vi "VisualizeModulePositioning_standalone.vi"() -> ()   [LabVIEW 2016]
uses:
  2_ModulePositioning/SingleModuleProgressReport.ctl
  <vilib>/vision/driver/NI_Vision_Acquisition_Software.lvlib
  <vilib>/vision/NI_Vision_Development_Module.lvlib
panel:
  in  "Placement tolerance [um]":dbl=10.0
  in  "Calibration [um/pix]":dbl=0.25
  out "delta Y":sgl
  out "delta X":sgl
  out "Current Position":T1
  in  "Axis Speeds":T2={"X [mm/s]"=25.0, "Y [mm/s]"=12.5, "Z [mm/s]"=5.0}
  in  "stop":bool
  out "Placement Monitor":T3(plugin-control)
  out "Fiducial Template":T3(plugin-control)
  in  "Templates path":path=path "C:/Users/Aerotech/Documents/BNL_ThermomechanicalStave"
  in  "Module fiducial marker":T4(ring)=enum."[None]"
  out "Module Progress Report":T5(array[cluster])
  in  "Camera Name":refnum<k21>="cam0" caption="IMAQdx Session"
  in  "N modules":i32
  in  "Calibrated positions of fiducials [mm]":dbl[][](array[numeric])=[[-675.4228165149058, -196.82430550413875, -11.55], [-579.8428201474238, -196.8506568257386, -11.55], [-579.816468825824, -101.27066045825673, -11.55], [-675.3964651933059, -101.24430913665685, -11.55], [-577.422820239396, -196.8513240176017, -11.55], [-481.84282387191405, -196.87767533920157, -11.55], [-481.8164725503142, -101.29767897171968, -11.55], [-577.396468917796, -101.2713276501198, -11.55], [-479.42282396388623, -196.87834253106465, -11.55], [-383.8428275964043, -196.90469385266454, -11.55], [-383.81647627480436, -101.32469748518264, -11.55], [-479.3964726422863, -101.29834616358275, -11.55], [-381.42282768837646, -196.90536104452758, -11.55], [-285.8428313208945, -196.93171236612747, -11.55], [-285.8164799992946, -101.35171599864559, -11.55], [-381.39647636677654, -101.3253646770457, -11.55], [-283.4228314128667, -196.93237955799054, -11.55], [-187.84283504538473, -196.95873087959043, -11.55], [-187.8164837237848, -101.37873451210854, -11.55], [-283.39648009126677, -101.35238319050865, -11.55], [-185.42283513735697, -196.9593980714535, -11.55], [-89.84283876987502, -196.98574939305337, -11.55], [-89.81648744827521, -101.40575302557149, -11.55], [-185.39648381575705, -101.3794017039716, -11.55], [-87.42283886184703, -196.98641658491644, -11.55], [8.157157505634814, -197.01276790651633, -11.55], [8.183508827234618, -101.43277153903443, -11.55], [-87.39648754024722, -101.40642021743454, -11.55], [10.57715741366269, -197.01343509837938, -11.55], [106.15715378114453, -197.0397864199793, -11.55], [106.18350510274433, -101.45979005249738, -11.55], [10.603508735262494, -101.4334387308975, -11.55], [108.57715368917252, -197.04045361184234, -11.55], [204.15715005665436, -197.06680493344223, -11.55], [204.18350137825416, -101.48680856596033, -11.55], [108.60350501077232, -101.46045724436046, -11.55], [206.57714996468223, -197.0674721253053, -11.55], [302.1571463321641, -197.09382344690516, -11.55], [302.1834976537639, -101.5138270794233, -11.55], [206.60350128628204, -101.4874757578234, -11.55], [304.57714624019206, -197.09449063876826, -11.55], [400.1571426076739, -197.12084196036813, -11.55], [400.1834939292737, -101.54084559288623, -11.55], [304.60349756179187, -101.51449427128635, -11.55], [402.5771425157018, -197.1215091522312, -11.55], [498.15713888318373, -197.1478604738311, -11.55], [498.18349020478354, -101.56786410634919, -11.55], [402.6034938373016, -101.5415127847493, -11.55], [500.5771387912116, -197.14852766569413, -11.55], [596.1571351586933, -197.17487898729405, -11.55], [596.1834864802931, -101.59488261981214, -11.55], [500.6034901128114, -101.56853129821225, -11.55]]
  # "-101.244"
  # "-196.851"
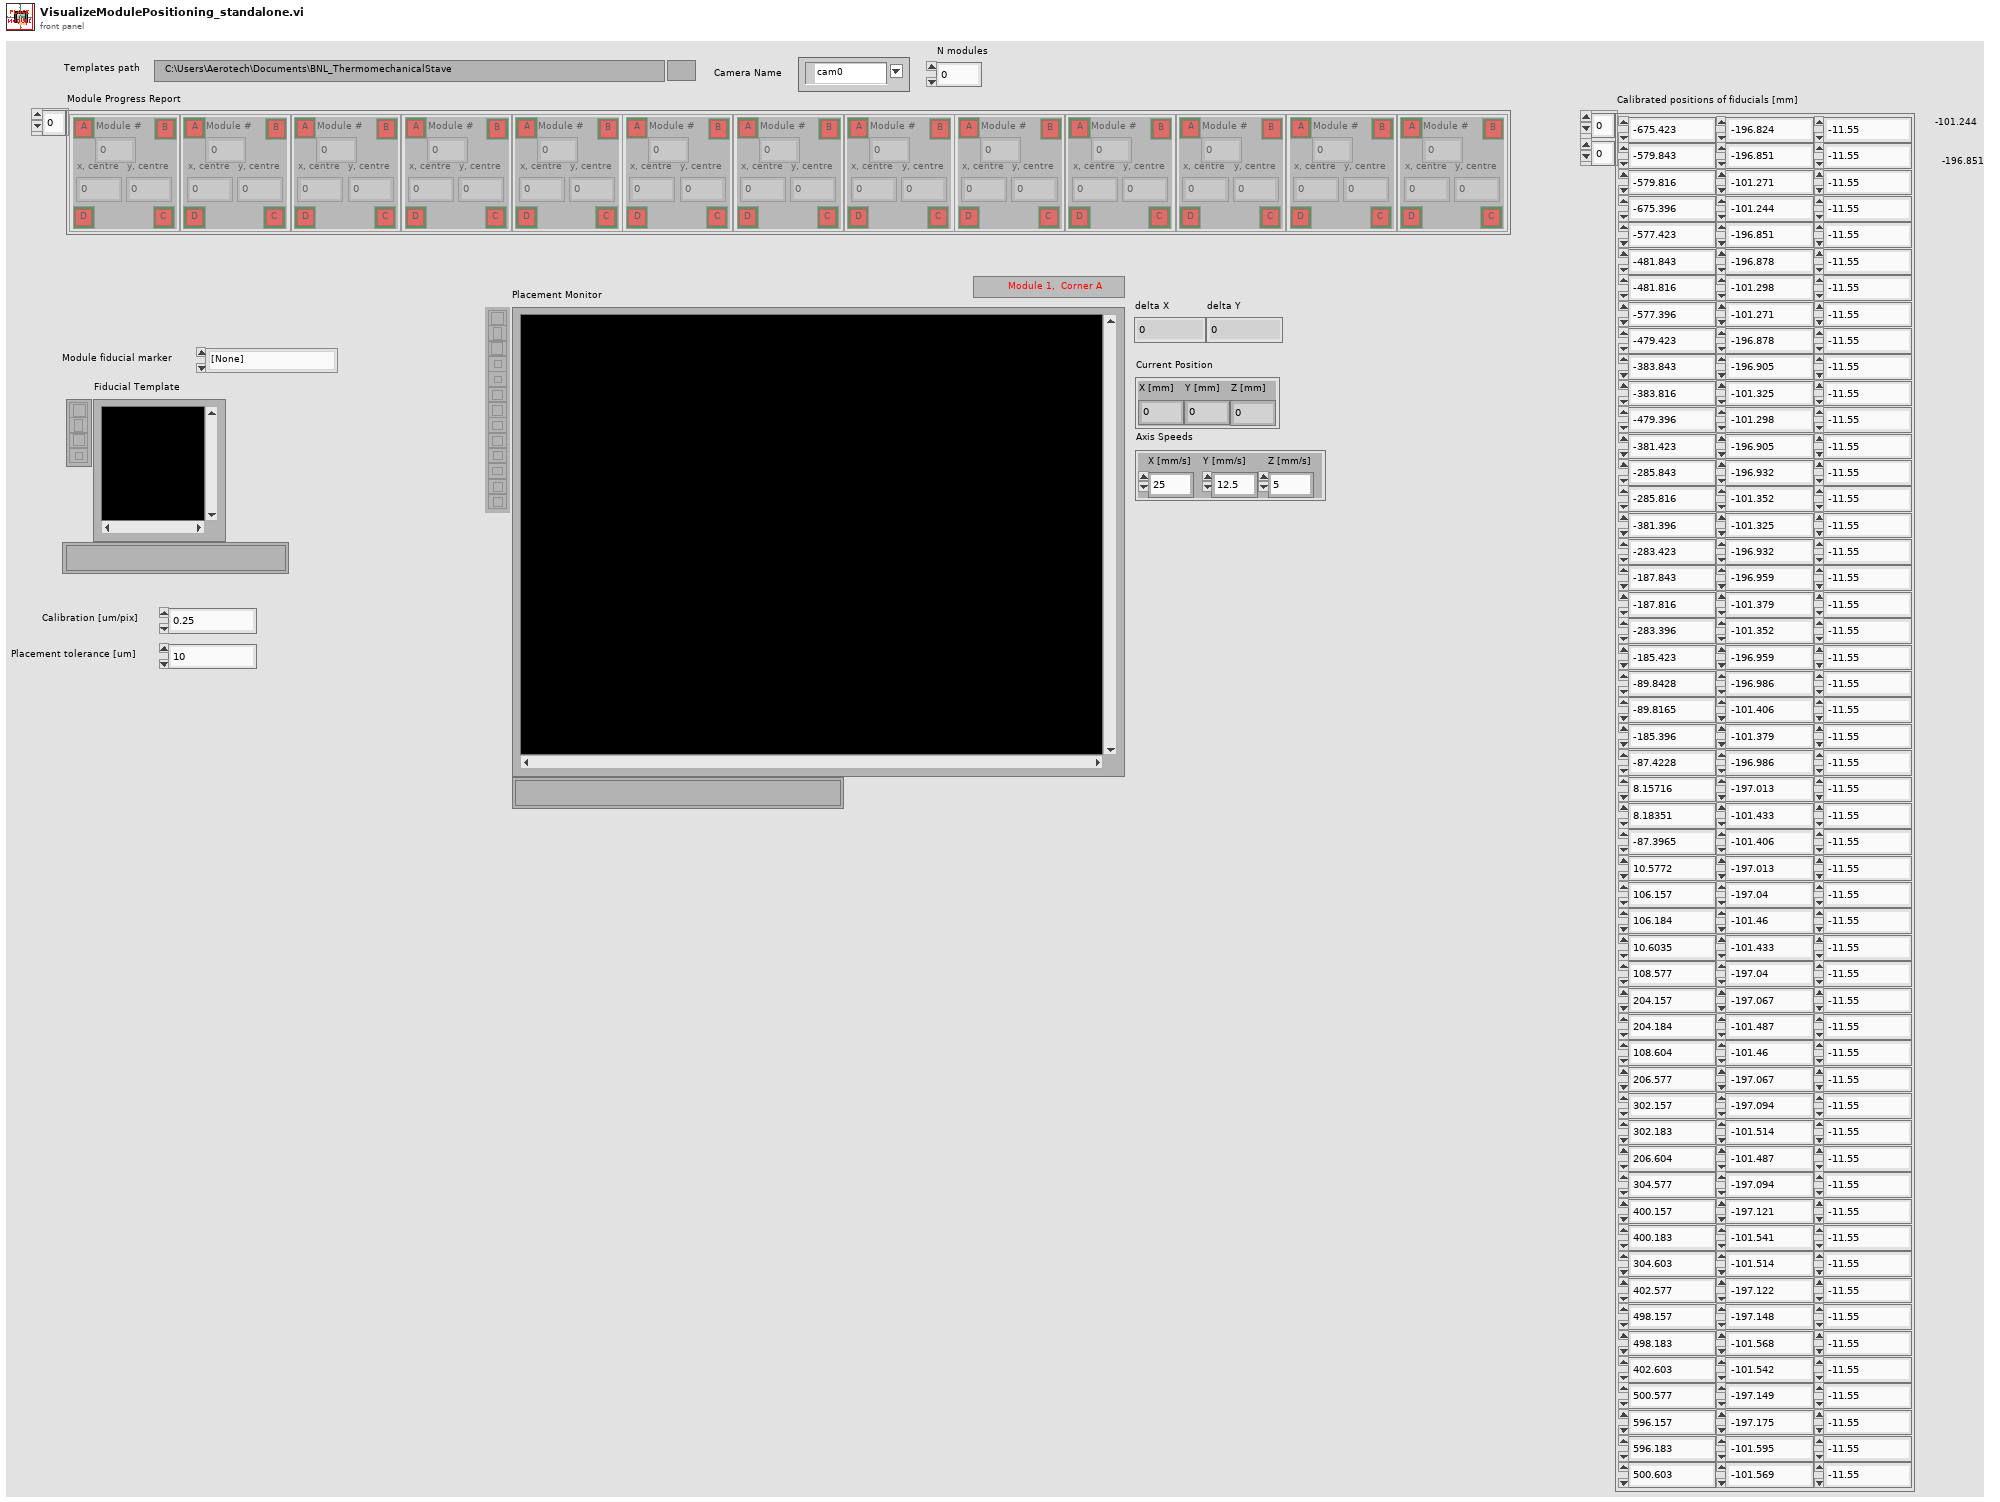
[diagram p1: front panel]
types:
  T1 = cluster{"X [mm]":dbl, "Y [mm]":dbl, "Z [mm]":dbl}
  T2 = cluster{"X [mm/s]":dbl, "Y [mm/s]":dbl, "Z [mm/s]":dbl}
  T3 = typedef "IMAQ Image.ctl" = refnum<image>
  T4 = enum16{"Mark C", "Mark B", "Strip Corner", "[None]"}
  T5 = cluster{"A":bool, "x, centre":dbl, "y, centre":dbl, "Module #":i32, "B":bool, "D":bool, "C":bool}[]
  T6 = typedef "SingleModuleProgressReport.ctl" = cluster{"A":bool, "x, centre":dbl, "y, centre":dbl, "Module #":i32, "B":bool, "D":bool, "C":bool}
  T7 = cluster{"Algorithm":i32, "Number of Matches Requested":i32, "Minimum Match Score":sgl, "SubPixel Accuracy":bool, "Rotation Angle Ranges":cluster{"Start":sgl, "End":sgl}[], "Show Search Area":bool, "Show Result":bool}
  T8 = typedef "IMAQdx.ctl" = refnum<k21>
  T9 = cluster{"Final X":dbl, "Final Y":dbl, "Final Z":dbl}
  T10 = cluster{"Position":cluster{"x":sgl, "y":sgl}, "Angle":sgl, "Scale":sgl, "Score":sgl, "Bounding Box":cluster{"x":sgl, "y":sgl}[]}[]
  T11 = cluster{"Position":cluster{"x":sgl, "y":sgl}, "Angle":sgl, "Scale":sgl, "Score":sgl, "Bounding Box":cluster{"x":sgl, "y":sgl}[]}
  T12 = cluster{"A":bool, "x, centre":dbl, "y, centre":dbl, "Module #":i32, "B":bool, "D":bool, "C":bool}
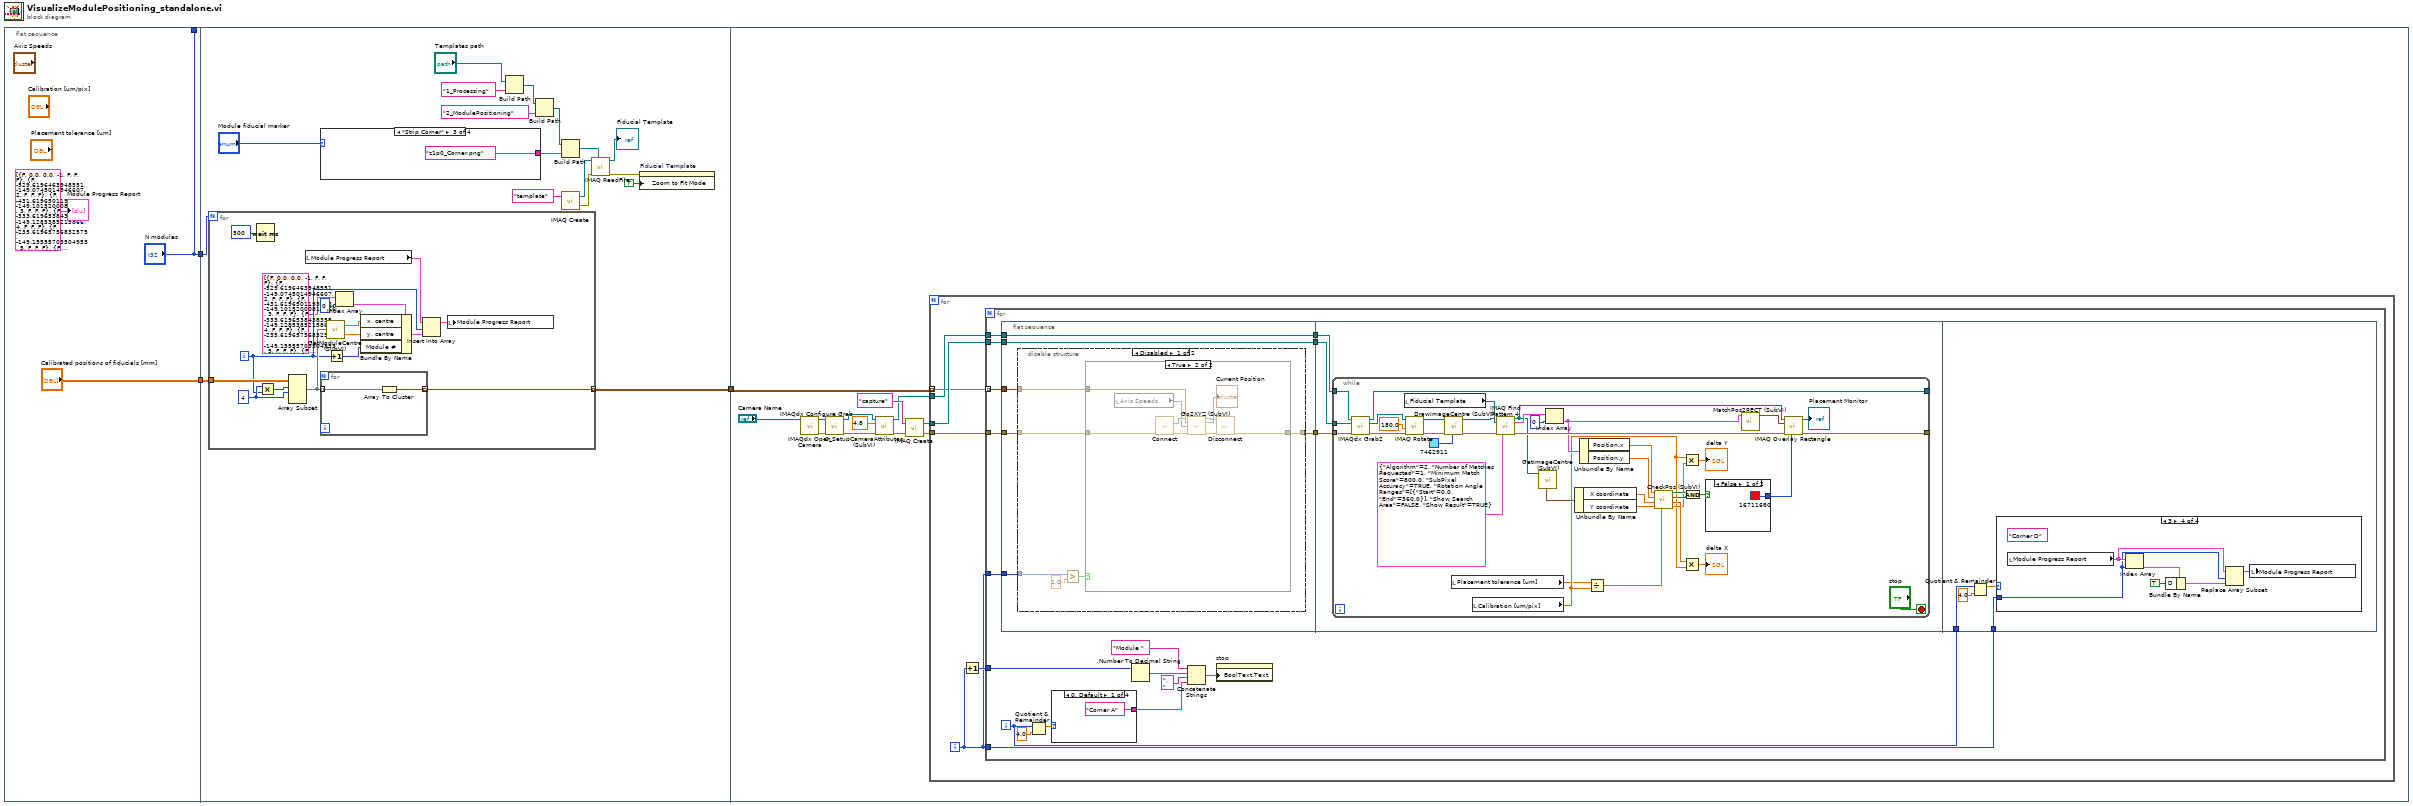
[diagram p0: block diagram]
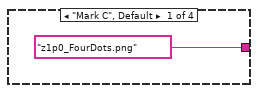
[diagram p2: hidden frame]
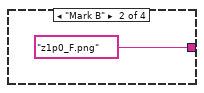
[diagram p3: hidden frame]
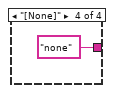
[diagram p4: hidden frame]
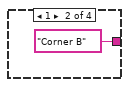
[diagram p5: hidden frame]
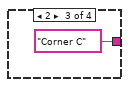
[diagram p6: hidden frame]
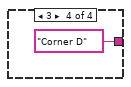
[diagram p7: hidden frame]
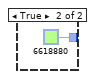
[diagram p10: hidden frame]
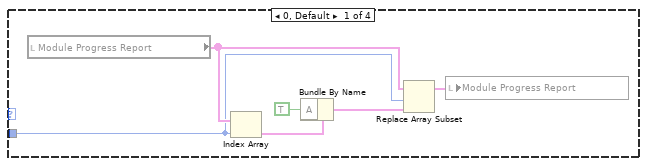
[diagram p11: hidden frame]
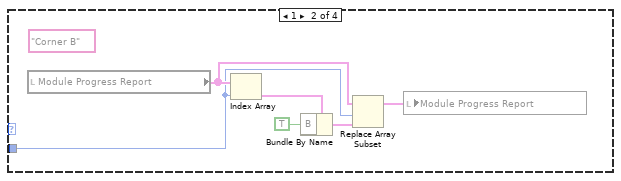
[diagram p12: hidden frame]
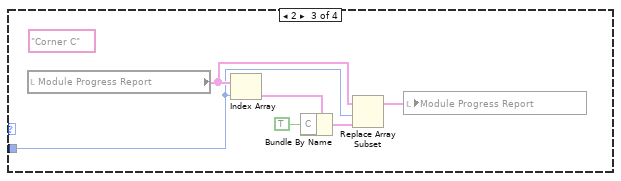
[diagram p13: hidden frame]
diagram:
  n1 = flat-sequence {
    tunnel: ["N modules"] -> _
    tunnel: ["N modules"] -> w2
    tunnel: ["Calibrated positions of fiducials [mm]"] -> w1
    tunnel: [w21] -> w3
    tunnel: w2 -> [w23]
    tunnel: w1 -> [w22]
    tunnel: w3 -> [w46]
    frame #0 {
      "Module Progress Report" <- T6[] [{"A"=FALSE, "x, centre"=0.0, "y, centre"=0.0, "Module #"=-1, "B"=FALSE, "D"=FALSE, "C"=FALSE}, {"A"=FALSE, "x, centre"=-529.6196463948551, "y, centre"=-149.0745014946607, "Module #"=2, "B"=FALSE, "D"=FALSE, "C"=FALSE}, {"A"=FALSE, "x, centre"=-431.6196501193453, "y, centre"=-149.10152000812366, "Module #"=3, "B"=FALSE, "D"=FALSE, "C"=FALSE}, {"A"=FALSE, "x, centre"=-333.6196538438355, "y, centre"=-149.1285385215866, "Module #"=4, "B"=FALSE, "D"=FALSE, "C"=FALSE}, {"A"=FALSE, "x, centre"=-235.61965756832575, "y, centre"=-149.15555703504953, "Module #"=5, "B"=FALSE, "D"=FALSE, "C"=FALSE}, {"A"=FALSE, "x, centre"=-137.6196612928161, "y, centre"=-149.1825755485125, "Module #"=6, "B"=FALSE, "D"=FALSE, "C"=FALSE}, {"A"=FALSE, "x, centre"=-627.6196426703649, "y, centre"=-149.04748298119773, "Module #"=1, "B"=FALSE, "D"=FALSE, "C"=FALSE}, {"A"=FALSE, "x, centre"=-529.6196463948551, "y, centre"=-149.0745014946607, "Module #"=2, "B"=FALSE, "D"=FALSE, "C"=FALSE}, {"A"=FALSE, "x, centre"=-431.6196501193453, "y, centre"=-149.10152000812366, "Module #"=3, "B"=FALSE, "D"=FALSE, "C"=FALSE}, {"A"=FALSE, "x, centre"=-333.6196538438355, "y, centre"=-149.1285385215866, "Module #"=4, "B"=FALSE, "D"=FALSE, "C"=FALSE}, {"A"=FALSE, "x, centre"=-235.61965756832575, "y, centre"=-149.15555703504953, "Module #"=5, "B"=FALSE, "D"=FALSE, "C"=FALSE}, {"A"=FALSE, "x, centre"=-137.6196612928161, "y, centre"=-149.1825755485125, "Module #"=6, "B"=FALSE, "D"=FALSE, "C"=FALSE}, {"A"=FALSE, "x, centre"=-39.619665017306204, "y, centre"=-149.20959406197545, "Module #"=7, "B"=FALSE, "D"=FALSE, "C"=FALSE}, {"A"=FALSE, "x, centre"=58.38033125820351, "y, centre"=-149.2366125754384, "Module #"=8, "B"=FALSE, "D"=FALSE, "C"=FALSE}, {"A"=FALSE, "x, centre"=156.38032753371334, "y, centre"=-149.26363108890132, "Module #"=9, "B"=FALSE, "D"=FALSE, "C"=FALSE}, {"A"=FALSE, "x, centre"=254.38032380922306, "y, centre"=-149.29064960236428, "Module #"=10, "B"=FALSE, "D"=FALSE, "C"=FALSE}, {"A"=FALSE, "x, centre"=352.3803200847329, "y, centre"=-149.31766811582725, "Module #"=11, "B"=FALSE, "D"=FALSE, "C"=FALSE}, {"A"=FALSE, "x, centre"=450.38031636024266, "y, centre"=-149.3446866292902, "Module #"=12, "B"=FALSE, "D"=FALSE, "C"=FALSE}, {"A"=FALSE, "x, centre"=548.3803126357524, "y, centre"=-149.37170514275314, "Module #"=13, "B"=FALSE, "D"=FALSE, "C"=FALSE}] ("Module Progress Report")
    }
    frame #1 {
      n2 = for {
        N: w23 -> [_]
        tunnel: w22 -> [w43]
        tunnel: [w40] -> w21 mode=indexing
        i -> [w31]
        w41 = 4 ("x")
        n3 = Wait (ms)(milliseconds to wait=u32 500) -> ()  [unwired: 1 out]
        n4 = Multiply(x=w41, y=w31) -> (x*y=w42:i32)
        n5 = Array Subset(array=w43, index (row)=w42, length (row)=w41) -> (w39:dbl[][])  [unwired: 2 in]
        n6 = local read "Module Progress Report"() -> (w32:T5)
        n7 = for {
          tunnel: w39 -> [w44] mode=indexing
          tunnel: [w45] -> w40 mode=indexing
          n8 = Array To Cluster(array=w44) -> (cluster=w45:cluster{"[0]":dbl, "[1]":dbl, "[2]":dbl})
        }
        n9 = call "GetModuleCentre (SubVI).vi"("4x3 Array of Fiducial Coordinates"=w39) -> ("x, centre"=w38:dbl, "y, centre"=w37:dbl)
        n10 = Increment(x=w31) -> (x+1=w36:i32)
        n11 = Index Array(array=T6[] [{"A"=FALSE, "x, centre"=0.0, "y, centre"=0.0, "Module #"=-1, "B"=FALSE, "D"=FALSE, "C"=FALSE}, {"A"=FALSE, "x, centre"=-529.6196463948551, "y, centre"=-149.0745014946607, "Module #"=2, "B"=FALSE, "D"=FALSE, "C"=FALSE}, {"A"=FALSE, "x, centre"=-431.6196501193453, "y, centre"=-149.10152000812366, "Module #"=3, "B"=FALSE, "D"=FALSE, "C"=FALSE}, {"A"=FALSE, "x, centre"=-333.6196538438355, "y, centre"=-149.1285385215866, "Module #"=4, "B"=FALSE, "D"=FALSE, "C"=FALSE}, {"A"=FALSE, "x, centre"=-235.61965756832575, "y, centre"=-149.15555703504953, "Module #"=5, "B"=FALSE, "D"=FALSE, "C"=FALSE}, {"A"=FALSE, "x, centre"=-137.6196612928161, "y, centre"=-149.1825755485125, "Module #"=6, "B"=FALSE, "D"=FALSE, "C"=FALSE}, {"A"=FALSE, "x, centre"=-627.6196426703649, "y, centre"=-149.04748298119773, "Module #"=1, "B"=FALSE, "D"=FALSE, "C"=FALSE}, {"A"=FALSE, "x, centre"=-529.6196463948551, "y, centre"=-149.0745014946607, "Module #"=2, "B"=FALSE, "D"=FALSE, "C"=FALSE}, {"A"=FALSE, "x, centre"=-431.6196501193453, "y, centre"=-149.10152000812366, "Module #"=3, "B"=FALSE, "D"=FALSE, "C"=FALSE}, {"A"=FALSE, "x, centre"=-333.6196538438355, "y, centre"=-149.1285385215866, "Module #"=4, "B"=FALSE, "D"=FALSE, "C"=FALSE}, {"A"=FALSE, "x, centre"=-235.61965756832575, "y, centre"=-149.15555703504953, "Module #"=5, "B"=FALSE, "D"=FALSE, "C"=FALSE}, {"A"=FALSE, "x, centre"=-137.6196612928161, "y, centre"=-149.1825755485125, "Module #"=6, "B"=FALSE, "D"=FALSE, "C"=FALSE}, {"A"=FALSE, "x, centre"=-39.619665017306204, "y, centre"=-149.20959406197545, "Module #"=7, "B"=FALSE, "D"=FALSE, "C"=FALSE}, {"A"=FALSE, "x, centre"=58.38033125820351, "y, centre"=-149.2366125754384, "Module #"=8, "B"=FALSE, "D"=FALSE, "C"=FALSE}, {"A"=FALSE, "x, centre"=156.38032753371334, "y, centre"=-149.26363108890132, "Module #"=9, "B"=FALSE, "D"=FALSE, "C"=FALSE}, {"A"=FALSE, "x, centre"=254.38032380922306, "y, centre"=-149.29064960236428, "Module #"=10, "B"=FALSE, "D"=FALSE, "C"=FALSE}, {"A"=FALSE, "x, centre"=352.3803200847329, "y, centre"=-149.31766811582725, "Module #"=11, "B"=FALSE, "D"=FALSE, "C"=FALSE}, {"A"=FALSE, "x, centre"=450.38031636024266, "y, centre"=-149.3446866292902, "Module #"=12, "B"=FALSE, "D"=FALSE, "C"=FALSE}, {"A"=FALSE, "x, centre"=548.3803126357524, "y, centre"=-149.37170514275314, "Module #"=13, "B"=FALSE, "D"=FALSE, "C"=FALSE}] ("Module Progress Report"), index=0) -> (element=w33:T6)
        n12 = Bundle By Name(cluster=w33, "x, centre"=w38, "y, centre"=w37, "Module #"=w36) -> (w28:T6)
        n13 = Insert Into Array(array=w32, index=w31, new element=w28) -> (w30:T5)
        n14 = local write "Module Progress Report"(w30) -> ()
      }
      n15 = case shown="\"Strip Corner\"" "Module fiducial marker" {
        tunnel: ["z1p0_FourDots.png" ("name or relative path") "z1p0_F.png" ("name or relative path") "z1p0_Corner.png" ("name or relative path") "none" ("name or relative path")] -> w20
        frame "Mark C", Default {
        }
        frame "Mark B" {
        }
        frame "Strip Corner" {
        }
        frame "[None]" {
        }
      }
      n16 = Build Path(base path="Templates path", name or relative path="1_Processing") -> (appended path=w7:path)
      n17 = Build Path(base path=w7, name or relative path="2_ModulePositioning") -> (appended path=w18:path)
      n18 = Build Path(base path=w18, name or relative path=w20) -> (appended path=w17:path)
      n19 = call "IMAQ Create"("Image Name"="template") -> ("New Image"=w16:T3, "error out"=w15:errorcluster)  [unwired: 4 in]
      n20 = call "IMAQ ReadFile"("File Path"=w17, "error in (no error)"=w15, "Image"=w16) -> ("error out"=w11:errorcluster, "Image Out"=→"Fiducial Template":T3)  [unwired: 4 in, 3 out]
      n21 = property on="Fiducial Template" class="ImageControl"(error in=w11, "Zoom to Fit Mode"=TRUE) -> ()  [unwired: 1 in, 2 out]
    }
    frame #2 {
      n22 = call <vilib>:"IMAQdx Open Camera.vi"("Session In"="Camera Name") -> ("error out"=w55:errorcluster, "Session Out"=w56:T8)  [unwired: 2 in, 7 out]
      n23 = call <vilib>:"IMAQdx Configure Grab.vi"("error in"=w55, "Session In"=w56) -> ("error out"=w53:errorcluster, "Session Out"=w54:T8)  [unwired: 8 out]
      n24 = call "0_SetupCameraAttributes (SubVI).vi"("error in (no error)"=w53, "Gain"=4.8, "Camera session in"=w54) -> ("error out"=w51:errorcluster, "Camera session out"=w48:T8)  [unwired: 7 in]
      n25 = call "IMAQ Create"("Image Name"="capture", "error in (no error)"=w51) -> ("New Image"=w49:T3, "error out"=w47:errorcluster)  [unwired: 3 in]
      n26 = for {
        tunnel: w48 -> [w63]
        tunnel: w49 -> [w62]
        tunnel: w47 -> [w61]
        tunnel: w46 -> [w59] mode=indexing
        i -> [w58]
        n27 = Increment(x=w58) -> (x+1=w60:i32)
        n28 = for {
          tunnel: w63 -> [w78]
          tunnel: w62 -> [w77]
          tunnel: w61 -> [w76]
          tunnel: w60 -> [w71]
          tunnel: w59 -> [w67] mode=indexing
          tunnel: w58 -> [w66]
          tunnel: w58 -> [w64]
          i -> [w65]
          n29 = flat-sequence {
            tunnel: w78 -> [w90]
            tunnel: w76 -> [w89]
            tunnel: w77 -> [w91]
            tunnel: [w91] -> w81
            tunnel: [w88] -> w80
            tunnel: [w90] -> w79
            tunnel: w67 -> [w87]
            tunnel: w64 -> [w86]
            tunnel: w81 -> [w110]
            tunnel: w80 -> [w109]
            tunnel: w79 -> [w108]
            tunnel: w66 -> [w153]
            tunnel: w65 -> [w152]
            frame #0 {
              n30 = disable-structure shown="Disabled" {
                disable-tunnel: w89 -> [w97 _]
                disable-tunnel: [w96 _] -> w88
                disable-tunnel: w87 -> [w95 _]
                disable-tunnel: w86 -> [w92 _]
                frame Disabled {
                  n31 = Greater?(x=w92, y=1.0) -> (0:w94:bool)
                  n32 = case shown="True" w94 {
                    tunnel: w97 -> [w98 w107]
                    tunnel: [w98 w106] -> w96
                    tunnel: w95 -> [_ w105]
                    frame False {
                      # "Temporarily skip corners C and D"
                    }
                    frame True {
                      n33 = local read "Axis Speeds"() -> (w99:T2)
                      n34 = call "Connect.vi"("error in (no error)"=w107) -> ("error out"=w103:errorcluster, "controller"=w102:refnum<k24>)  [unwired: 9 in]
                      n35 = call "Go2XYZ (SubVI).vi"(".NET Refnum in"=w102, "Go to Coordinates"=w105, "Axis Speeds"=w99, "error in (no error)"=w103) -> (".NET Refnum out"=w101:refnum<k24>, "Final Position"=→"Current Position":T9, "error out"=w100:errorcluster)  [unwired: 7 in, 2 out]
                      n36 = call "Disconnect.vi"("error in (no error)"=w100, "controller"=w101) -> ("error out"=w106:errorcluster)  [unwired: 9 in]
                    }
                  }
                }
                frame Enabled {
                }
              }
            }
            frame #1 {
              n37 = while {
                tunnel: w110 -> [w149]
                tunnel: w109 -> [w148]
                tunnel: w108 -> [w147]
                tunnel: [w143] -> _
                tunnel: [w135] -> _
                stop <- "stop" stop-if-true
                n38 = call <vilib>:"IMAQdx Grab2.vi"("error in"=w148, "Image In"=w149, "Session In"=w147) -> ("error out"=w144:errorcluster, "Image Out"=w146:T3, "Session Out"=w143:T8)  [unwired: 5 in, 1 out]
                n39 = local read "Fiducial Template"() -> (w140:T3)
                n40 = call "IMAQ Rotate"("error in (no error)"=w144, "Angle (degrees)"=sgl 180.0, "Image Src"=w146) -> ("error out"=w116:errorcluster, "Image Dst Out"=w118:T3)  [unwired: 7 in]
                n41 = call "DrawImageCentre (SubVI).vi"("Axis colour"=u32 7462911, "error in (no error)"=w116, "Refnum in"=w118) -> ("error out"=w115:errorcluster, "Refnum out"=w117:T3)  [unwired: 7 in]
                n42 = local read "Placement tolerance [um]"() -> (w111:dbl)
                n43 = local read "Calibration [um/pix]"() -> (w112:dbl)
                n44 = call "IMAQ Find Pattern 4"("Image"=w117, "Template"=w140, "error in"=w115, "Settings"=T7 {"Algorithm"=2, "Number of Matches Requested"=1, "Minimum Match Score"=800.0, "SubPixel Accuracy"=TRUE, "Rotation Angle Ranges"=[{"Start"=0.0, "End"=360.0}], "Show Search Area"=FALSE, "Show Result"=TRUE}) -> ("Image Out"=w129:T3, "Matches (pixel)"=w138:T10, "error out"=w136:errorcluster)  [unwired: 5 in, 4 out]
                n45 = call "GetImageCentre (SubVI).vi"("Image in \n(refnum)"=w129) -> ("Centre Point"=w128:cluster{"X coordinate":dbl, "Y coordinate":dbl})  [unwired: 4 in, 4 out]
                n46 = Index Array(array=w138, index=0) -> (element=w123:T11)
                n47 = Unbundle By Name(w128) -> ("X coordinate"=w127:dbl, "Y coordinate"=w126:dbl)
                n48 = Unbundle By Name(w123) -> ("Position.x"=w133:sgl, "Position.y"=w132:sgl)
                n49 = Divide(x=w111, y=w112) -> (x/y=w113:dbl)
                n50 = call "CheckPos (SubVI).vi"("x"=w133, "y"=w132, "true x"=w127, "true y"=w126, "variation tolerance"=w113) -> ("pass x coordinate"=w131:bool, "pass y coordinate"=w130:bool, "delta X"=w122:sgl, "delta Y"=w121:sgl)  [unwired: 2 in]
                n51 = Multiply(x=w112, y=w121) -> (x*y=→"delta Y":dbl)
                n52 = Multiply(x=w122, y=w112) -> (x*y=→"delta X":dbl)
                n53 = And(x=w131, y=w130) -> (x .and. y?=w125:bool)
                n54 = case shown="False" w125 {
                  tunnel: [u32 16711680 ("Color") u32 6618880 ("Color")] -> w124
                  frame False {
                  }
                  frame True {
                  }
                }
                n55 = call "MatchPos2RECT (SubVI).vi"("Match element"=w123) -> ("Rectangle"=w139:cluster{"x":sgl, "y":sgl, dbl, dbl})  [unwired: 10 in]
                n56 = call "IMAQ Overlay Rectangle"("Color"=w124, "error in (no error)"=w136, "Rectangle"=w139, "Image"=w129) -> ("error out"=w135:errorcluster, "Image Out"=→"Placement Monitor":T3)  [unwired: 6 in]
              }
            }
            frame #2 {
              n57 = Quotient & Remainder(x=w152, y=4.0) -> (x-y*floor(x/y)=w155:dbl)  [unwired: 1 out]
              n58 = case shown="3" w155 {
                tunnel: w153 -> [w158 w162 w168 w174]
                frame 0, Default {
                  n59 = local read "Module Progress Report"() -> (w159:T5)
                  n60 = Index Array(array=w159, index=w158) -> (element=w157:T12)
                  n61 = Bundle By Name(cluster=w157, "A"=TRUE) -> (w160:T12)
                  n62 = Replace Array Subset(array=w159, new element=w160, index=w158) -> (w156:T5)
                  n63 = local write "Module Progress Report"(w156) -> ()
                }
                frame 1 {
                  (unwired) "Corner B"
                  n64 = local read "Module Progress Report"() -> (w165:T5)
                  n65 = Index Array(array=w165, index=w162) -> (element=w164:T12)
                  n66 = Bundle By Name(cluster=w164, "B"=TRUE ("A")) -> (w166:T12)
                  n67 = Replace Array Subset(array=w165, new element=w166, index=w162) -> (w163:T5)
                  n68 = local write "Module Progress Report"(w163) -> ()
                }
                frame 2 {
                  (unwired) "Corner C"
                  n69 = local read "Module Progress Report"() -> (w171:T5)
                  n70 = Index Array(array=w171, index=w168) -> (element=w170:T12)
                  n71 = Bundle By Name(cluster=w170, "C"=TRUE ("A")) -> (w172:T12)
                  n72 = Replace Array Subset(array=w171, new element=w172, index=w168) -> (w169:T5)
                  n73 = local write "Module Progress Report"(w169) -> ()
                }
                frame 3 {
                  (unwired) "Corner D"
                  n74 = local read "Module Progress Report"() -> (w177:T5)
                  n75 = Index Array(array=w177, index=w174) -> (element=w176:T12)
                  n76 = Bundle By Name(cluster=w176, "D"=TRUE ("A")) -> (w178:T12)
                  n77 = Replace Array Subset(array=w177, new element=w178, index=w174) -> (w175:T5)
                  n78 = local write "Module Progress Report"(w175) -> ()
                }
              }
            }
          }
          n79 = Quotient & Remainder(x=w65, y=4.0) -> (x-y*floor(x/y)=w68:dbl)  [unwired: 1 out]
          n80 = case shown="0, Default" w68 {
            tunnel: ["Corner A" "Corner B" "Corner C" "Corner D"] -> w70
            frame 0, Default {
            }
            frame 1 {
            }
            frame 2 {
            }
            frame 3 {
            }
          }
          n81 = Number To Decimal String(number=w71) -> (decimal integer string=w74:string)  [unwired: 1 in]
          n82 = Concatenate Strings("Module " ("string"), w74, ",  " ("string"), w70) -> (w75:string)
          n83 = property on="stop" class="Bool"("BoolText.Text"=w75) -> ()  [unwired: 2 in, 2 out]
        }
      }
    }
  }
